vi "VA CoAP - Server - Proccess Message - Gets Value from JSON.vi"(8 "error in (no error)":errorcluster, 10 "Item name":string[](array[string]), 11 "JSON Value in":refnum<class "JSON Value.lvclass">) -> (0 "error out":errorcluster, 2 "Value":string, 3 "JSON Value out":refnum<class "JSON Value.lvclass">)   [LabVIEW 2020]
uses:
  <vilib>/addons/JSON API/JSON Value/JSON Value.lvclass
  <vilib>/addons/JSON API/JSON Value/Get as JSON string (pretty).vi
  <vilib>/addons/JSON API/Get Polymorphic/JSON GetSet.lvlib
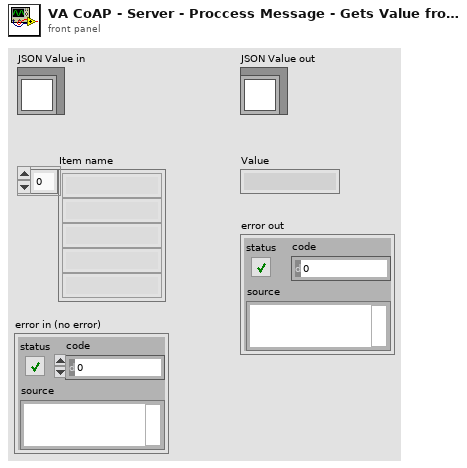
[diagram p1: front panel]
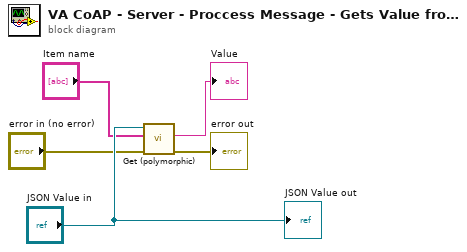
[diagram p0: block diagram]
diagram:
  n1 = call-poly <vilib>:"Get (polymorphic).vi"("error in (no error)"="error in (no error)", "Name Array"="Item name", "JSON Value in"="JSON Value in") -> ("error out"=→"error out":errorcluster, "<JSON>"=→"Value":string)  [unwired: 7 in]
  "JSON Value out" <- "JSON Value in"
